vi "SnoLaunchesCatapult[Conflict 1].vi"   [LabVIEW 2013]
uses:
  <vilib>/Rock Robotics/WPI/Solenoid/WPI_SolenoidValue.ctl
  <vilib>/Rock Robotics/WPI/Solenoid/WPI_SolenoidSetEnum.vi
types:
  T1 = typedef "WPI_SolenoidValue.ctl" = enum16{"Off", "On", "Forward", "Reverse"}
  T2 = typedef "WPI_SolenoidDevRef.ctl" = cluster{"DevStatus":errorcluster, "Solenoid Module":T3, "Forward Solenoid Channel":T4, "Reverse Solenoid Channel":T4}
  T3 = typedef "FPGA_TypedefSolenoidModule.ctl" = enum16{"Solenoid Module 1", "Solenoid Module 2"}
  T4 = typedef "WPI_SolenoidChannel.ctl" = enum8{"Solenoid 1", "Solenoid 2", "Solenoid 3", "Solenoid 4", "Solenoid 5", "Solenoid 6", "Solenoid 7", "Solenoid 8", "Invalid"}
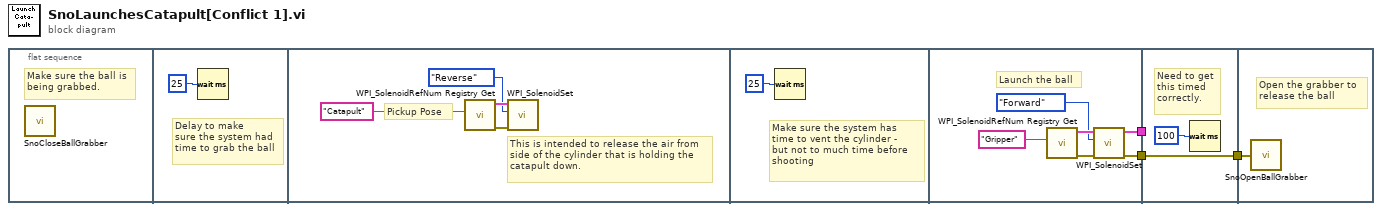
[diagram p0: block diagram]
diagram:
  n1 = flat-sequence {
    tunnel: [w11] -> w3
    tunnel: [w10] -> w2
    tunnel: w3 -> [_]
    tunnel: w2 -> [w16]
    tunnel: [w16] -> w1
    tunnel: w1 -> [w18]
    frame #0 {
      # "Make sure the ball is\nbeing grabbed."
      n2 = call "SnoCloseBallGrabber.vi"() -> ()  [unwired: 1 in, 2 out]
    }
    frame #1 {
      # "Delay to make\nsure the system had\ntime to grab the ball"
      n3 = Wait (ms)(milliseconds to wait=u32 25) -> ()  [unwired: 1 out]
    }
    frame #2 {
      # "This is intended to release the air from\nside of the cylinder that is holding the\ncatapult down."
      # "Pickup Pose"
      n4 = call <vilib>:"WPI_SolenoidRefNum Registry Get.vi"("refnum name"="Catapult") -> ("error out"=w8:errorcluster, "SolenoidDevRef"=w7:T2)  [unwired: 9 in]
      n5 = call-poly <vilib>:"WPI_SolenoidSet.vi"("error in (no error)"=w8, "Value"=WPI_SolenoidValue."Reverse", "SolenoidDevRef"=w7) -> ()  [unwired: 7 in, 2 out]
    }
    frame #3 {
      # "Make sure the system has\ntime to vent the cylinder -\nbut not to much time before\nshooting"
      n6 = Wait (ms)(milliseconds to wait=u32 25) -> ()  [unwired: 1 out]
    }
    frame #4 {
      # "Launch the ball"
      n7 = call <vilib>:"WPI_SolenoidRefNum Registry Get.vi"("refnum name"="Gripper") -> ("error out"=w14:errorcluster, "SolenoidDevRef"=w15:T2)  [unwired: 9 in]
      n8 = call-poly <vilib>:"WPI_SolenoidSet.vi"("error in (no error)"=w14, "Value"=WPI_SolenoidValue."Forward", "SolenoidDevRef"=w15) -> ("error out"=w10:errorcluster, "SolenoidDevRef"=w11:T2)  [unwired: 7 in]
    }
    frame #5 {
      # "Need to get\nthis timed\ncorrectly."
      n9 = Wait (ms)(milliseconds to wait=u32 100) -> ()  [unwired: 1 out]
    }
    frame #6 {
      # "Open the grabber to\nrelease the ball"
      n10 = call "SnoOpenBallGrabber.vi"("Input Error"=w18) -> ()  [unwired: 1 out]
    }
  }
